vi "FTT-main.vi"() -> ()   [LabVIEW 2014]
uses:
  global variable.vi
panel:
  in  "开始":bool
  in  "Line name":string="RO1"
  in  "Target":dbl
  in  "Plan":dbl
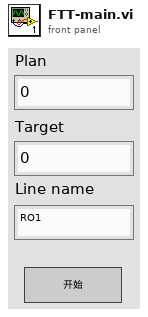
[diagram p1: front panel]
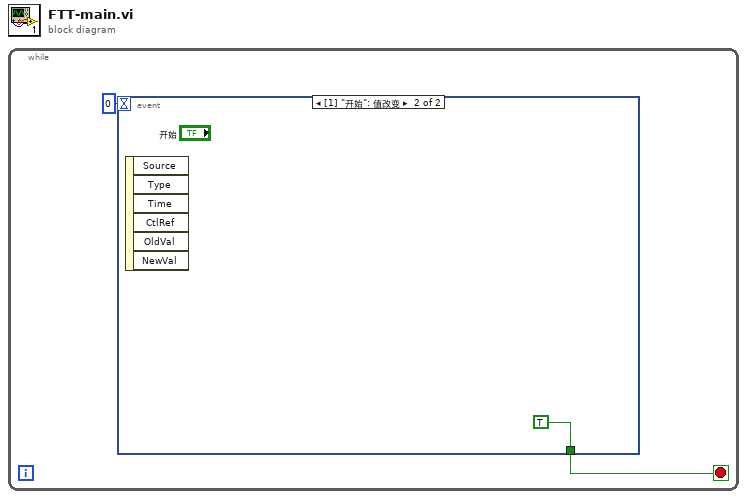
[diagram p0: block diagram]
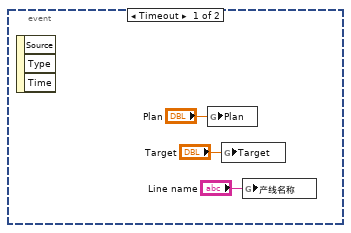
[diagram p2: hidden frame]
diagram:
  n1 = while {
    stop <- w1 stop-if-true
    n2 = event shown="[1] \"开始\": 值改变" {
      selector: _ -> [_ _]
      dyn-events: _ -> [_ _]
      timeout: 0 -> [_ _]
      tunnel: [_ TRUE] -> w1
      event Timeout {
        n3 = event-data() -> ()  [unwired: 1 in, 3 out]
        n4 = global write "global variable.vi" "Plan"("Plan") -> ()
        n5 = global write "global variable.vi" "Target"("Target") -> ()
        n6 = global write "global variable.vi" "产线名称"("Line name") -> ()
      }
      event "开始": Value Change {
        n7 = event-data() -> ()  [unwired: 1 in, 6 out]
      }
    }
  }
